vi "FPGANic.Read-Debug-FIFOs.vi"(7 "Enabled FIFOs":T1, 8 "error in":errorcluster, 9 "Timeout":i32=80 format="%.0x", 10 "Clear Debug FIFOs":bool, 11 "FPGA VI Reference In":refnum<k20>) -> (0 "error out":errorcluster, 3 "Debug Data":T2)   [LabVIEW 2018]
uses:
  <vilib>/Utility/error.llb/Error Cluster From Error Code.vi
  <vilib>/rvi/errors/niLvFpgaAdjustHostInterfaceError.vi
  <vilib>/Field R&D Services/Logger/Private/Manager.vi
  <vilib>/rvi/interface/nirviMethod/nirviMethod.xnode
  <vilib>/FPGAPlugInAG/Dynamic/niLvFpga_ReadFifo_Dynamic.vi
  <vilib>/rvi/errors/niLvFpgaMergeErrorWithErrorCode.vi
  <vilib>/Field R&D Services/Logger/Logger.lvlib
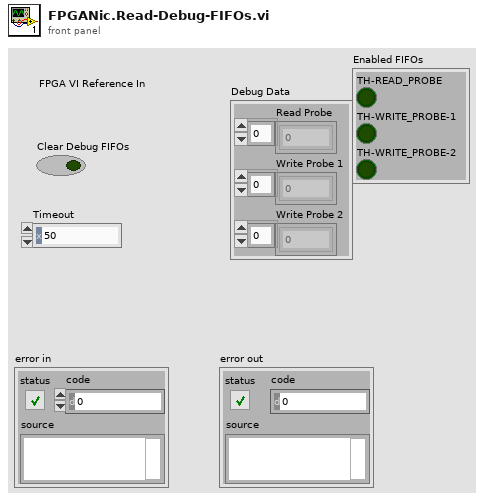
[diagram p1: front panel]
types:
  T1 = cluster{"TH-READ_PROBE":bool, "TH-WRITE_PROBE-1":bool, "TH-WRITE_PROBE-2":bool}
  T2 = cluster{"Read Probe":u64[], "Write Probe 1":u64[], "Write Probe 2":u64[]}
  T3 = cluster{"Data":u64[], "Data":u64[], "Data":u64[]}
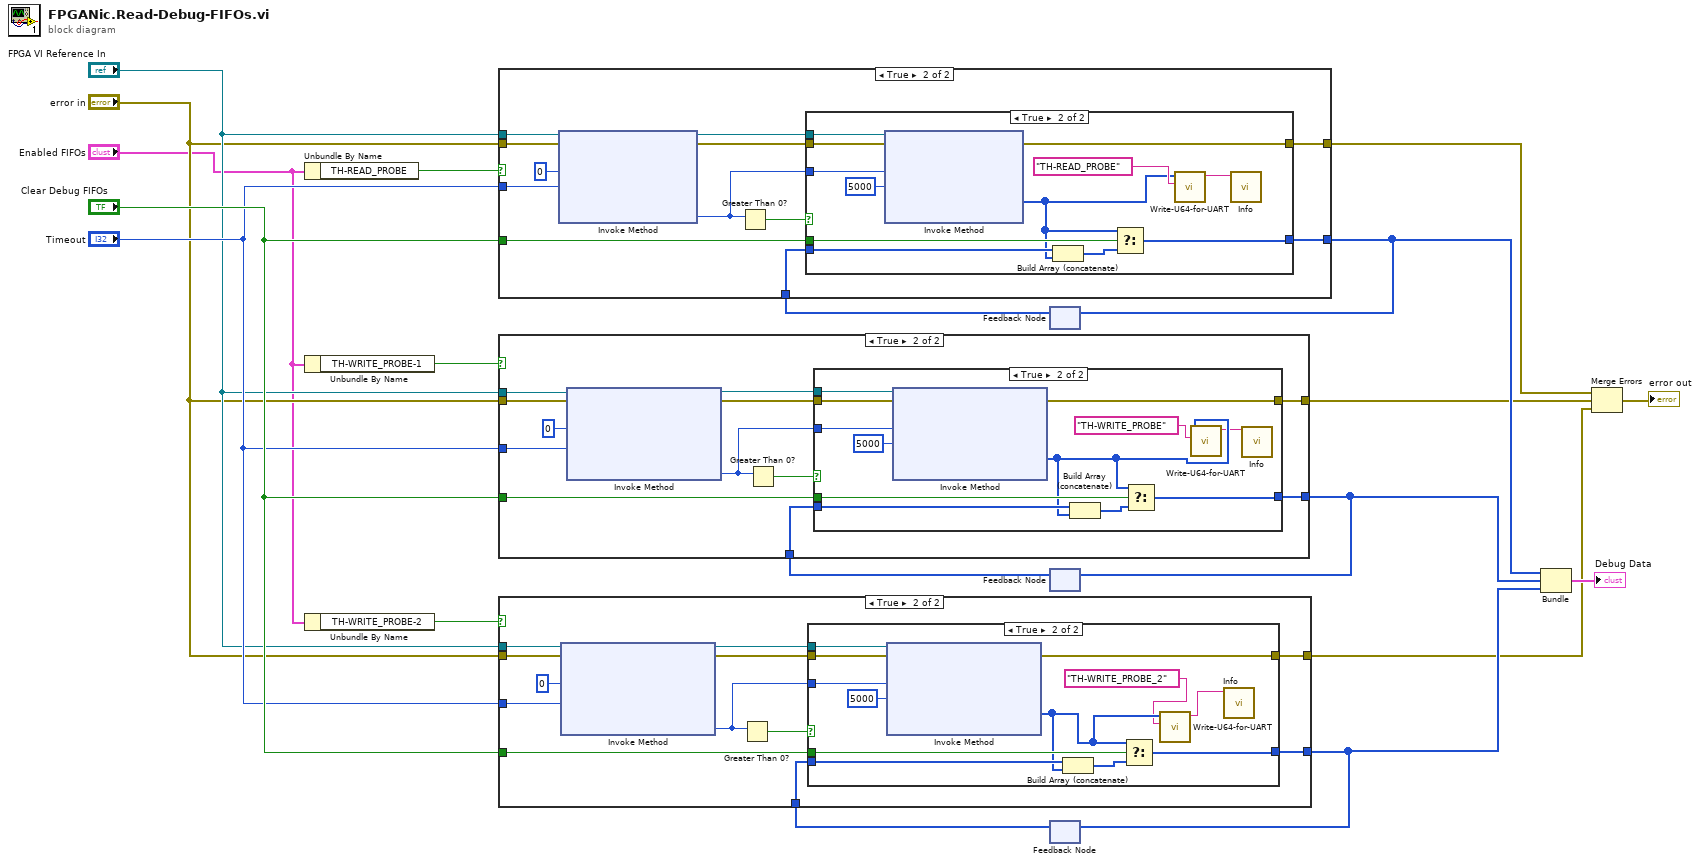
[diagram p0: block diagram]
diagram:
  n1 = Unbundle By Name("Enabled FIFOs") -> ("TH-READ_PROBE"=w9:bool)
  n2 = Unbundle By Name("Enabled FIFOs") -> ("TH-WRITE_PROBE-1"=w6:bool)
  n3 = Unbundle By Name("Enabled FIFOs") -> ("TH-WRITE_PROBE-2"=w5:bool)
  n4 = feedback #1() -> (w8:u64[])  [unwired: 1 in]
  n5 = case shown="True" w9 {
    tunnel: [w21 w28] -> w7
    tunnel: "Clear Debug FIFOs" -> [_ w27]
    tunnel: "Timeout" -> [_ w26]
    tunnel: "FPGA VI Reference In" -> [_ w25]
    tunnel: "error in" -> [w20 w24]
    tunnel: w8 -> [w21 w23]
    tunnel: [w20 w22] -> w4
    frame False {
    }
    frame True {
      n6 = xnode "Invoke Method"("FPGA VI Reference In"=w25, "error in"=w24, "Number of Elements"=u32 0, "Timeout (ms)"=w26) -> ("FPGA VI Reference Out"=w33:refnum<k20>, "error out"=w32:errorcluster, "Elements Remaining"=w31:u32)  [unwired: 1 out]
      n7 = Greater Than 0?(x=w31) -> (x > 0?=w30:bool)
      n8 = case shown="True" w30 {
        tunnel: w23 -> [w35 w47]
        tunnel: w31 -> [_ w46]
        tunnel: w32 -> [w34 w44]
        tunnel: w33 -> [_ w43]
        tunnel: [w35 w40] -> w28
        tunnel: [w34 w42] -> w22
        tunnel: w27 -> [_ w39]
        frame False {
        }
        frame True {
          n9 = xnode "Invoke Method"("FPGA VI Reference In"=w43, "error in"=w44, "Number of Elements"=w46, "Timeout (ms)"=5000) -> ("error out"=w42:errorcluster, "Data"=w37:u64[])  [unwired: 2 out]
          n10 = Build Array (concatenate)(w47, w37) -> (w41:u64[])
          n11 = Select(t=w37, s=w39, f=w41) -> (s? t:f=w40:u64[])
          n12 = call "Write-U64-for-UART.vi"("Log Message"="TH-READ_PROBE" ("string"), "Data"=w37) -> ("concatenated string"=w36:string)  [unwired: 9 in]
          n13 = call <vilib>:"Info.vi"("Message"=w36) -> ()  [unwired: 10 in, 1 out]
        }
      }
    }
  }
  n14 = feedback-in #1(w7) -> ()
  n15 = feedback #2() -> (w18:u64[])  [unwired: 1 in]
  n16 = case shown="True" w6 {
    tunnel: w18 -> [w49 w61]
    tunnel: "Clear Debug FIFOs" -> [_ w55]
    tunnel: [w49 w54] -> w14
    tunnel: "Timeout" -> [_ w53]
    tunnel: "FPGA VI Reference In" -> [_ w52]
    tunnel: "error in" -> [w48 w51]
    tunnel: [w48 w50] -> w3
    frame False {
    }
    frame True {
      n17 = xnode "Invoke Method"("FPGA VI Reference In"=w52, "error in"=w51, "Number of Elements"=u32 0, "Timeout (ms)"=w53) -> ("FPGA VI Reference Out"=w60:refnum<k20>, "error out"=w59:errorcluster, "Elements Remaining"=w58:u32)  [unwired: 1 out]
      n18 = Greater Than 0?(x=w58) -> (x > 0?=w57:bool)
      n19 = case shown="True" w57 {
        tunnel: w61 -> [w63 w75]
        tunnel: w58 -> [_ w74]
        tunnel: w59 -> [w62 w72]
        tunnel: w60 -> [_ w71]
        tunnel: [w63 w68] -> w54
        tunnel: [w62 w70] -> w50
        tunnel: w55 -> [_ w67]
        frame False {
        }
        frame True {
          n20 = xnode "Invoke Method"("FPGA VI Reference In"=w71, "error in"=w72, "Number of Elements"=w74, "Timeout (ms)"=5000) -> ("error out"=w70:errorcluster, "Data"=w65:u64[])  [unwired: 2 out]
          n21 = Build Array (concatenate)(w75, w65) -> (w69:u64[])
          n22 = Select(t=w65, s=w67, f=w69) -> (s? t:f=w68:u64[])
          n23 = call "Write-U64-for-UART.vi"("Log Message"="TH-WRITE_PROBE" ("string"), "Data"=w65) -> ("concatenated string"=w64:string)  [unwired: 9 in]
          n24 = call <vilib>:"Info.vi"("Message"=w64) -> ()  [unwired: 10 in, 1 out]
        }
      }
    }
  }
  n25 = feedback-in #2(w14) -> ()
  n26 = feedback #3() -> (w19:u64[])  [unwired: 1 in]
  n27 = case shown="True" w5 {
    tunnel: w19 -> [w76 w89]
    tunnel: [w76 w83] -> w17
    tunnel: "Clear Debug FIFOs" -> [_ w82]
    tunnel: "Timeout" -> [_ w81]
    tunnel: [w77 w80] -> w2
    tunnel: "FPGA VI Reference In" -> [_ w79]
    tunnel: "error in" -> [w77 w78]
    frame False {
    }
    frame True {
      n28 = xnode "Invoke Method"("FPGA VI Reference In"=w79, "error in"=w78, "Number of Elements"=u32 0, "Timeout (ms)"=w81) -> ("FPGA VI Reference Out"=w88:refnum<k20>, "error out"=w87:errorcluster, "Elements Remaining"=w86:u32)  [unwired: 1 out]
      n29 = Greater Than 0?(x=w86) -> (x > 0?=w85:bool)
      n30 = case shown="True" w85 {
        tunnel: w89 -> [w91 w103]
        tunnel: w86 -> [_ w102]
        tunnel: w87 -> [w90 w100]
        tunnel: w88 -> [_ w99]
        tunnel: [w91 w96] -> w83
        tunnel: [w90 w98] -> w80
        tunnel: w82 -> [_ w95]
        frame False {
        }
        frame True {
          n31 = xnode "Invoke Method"("FPGA VI Reference In"=w99, "error in"=w100, "Number of Elements"=w102, "Timeout (ms)"=5000) -> ("error out"=w98:errorcluster, "Data"=w94:u64[])  [unwired: 2 out]
          n32 = Build Array (concatenate)(w103, w94) -> (w97:u64[])
          n33 = Select(t=w94, s=w95, f=w97) -> (s? t:f=w96:u64[])
          n34 = call "Write-U64-for-UART.vi"("Log Message"="TH-WRITE_PROBE_2" ("string"), "Data"=w94) -> ("concatenated string"=w92:string)  [unwired: 9 in]
          n35 = call <vilib>:"Info.vi"("Message"=w92) -> ()  [unwired: 10 in, 1 out]
        }
      }
    }
  }
  n36 = feedback-in #3(w17) -> ()
  n37 = Bundle("Data"=w7, "Data"=w14, "Data"=w17) -> (→"Debug Data":T3)  [unwired: 1 in]
  n38 = Merge Errors(w4, w3, w2) -> (→"error out":errorcluster)
